vi "LoadGasCalibr.vi"(6 "Enable":bool, 7 "Read":bool, 8 "error in (no error)":errorcluster, 10 "Cluster":T1, 11 "VISA Refnum in":refnum<visa-resource-name>) -> (0 "error out":errorcluster, 1 "Array Graph":cluster{u16[], u16[]}[](array[cluster]), 3 "Array INT":i32[][](array[numeric]))   [LabVIEW 2020]
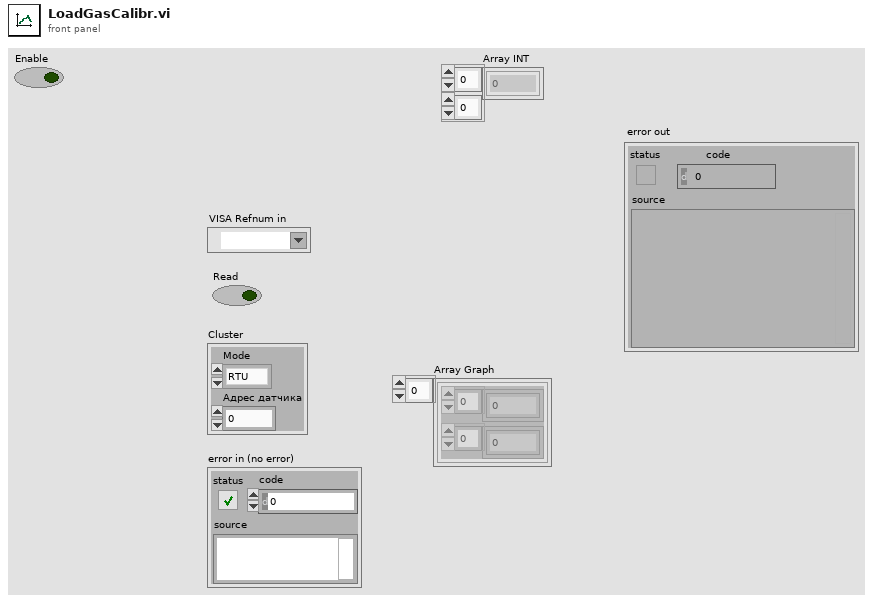
[diagram p1: front panel]
types:
  T1 = cluster{"Mode":enum16{"RTU", "ASCII"}, "Адрес датчика":u16}
  T2 = cluster{"Mode":enum16{"RTU", "ASCII"}, "Новый адрес датчика":u16}
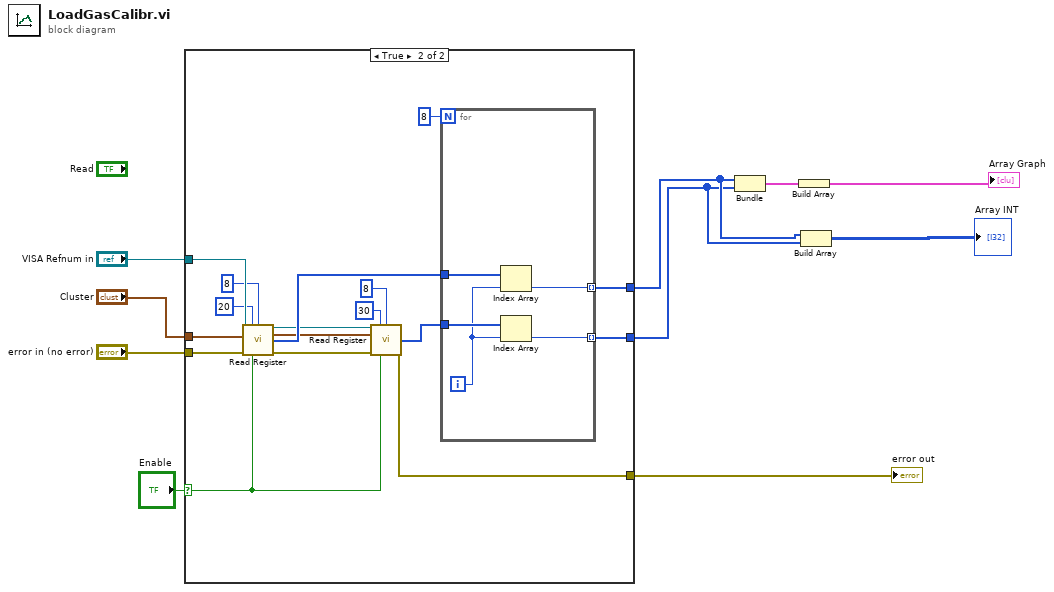
[diagram p0: block diagram]
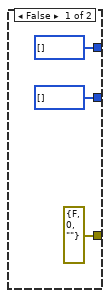
[diagram p2: hidden frame]
diagram:
  n1 = case shown="True" "Enable" {
    selector: "Enable" -> [_ w14]
    tunnel: "error in (no error)" -> [_ w24]
    tunnel: "Cluster" -> [_ w23]
    tunnel: "VISA Refnum in" -> [_ w22]
    tunnel: [errorcluster {"status"=FALSE, "code"=0, "source"=""} ("error out") w21] -> w6
    tunnel: [i32[] [] w16] -> w4
    tunnel: [i32[] [] w15] -> w3
    frame False {
    }
    frame True {
      n2 = call "Read Register.vi"("Refnum in"=w22, "startReg"=20 ("x"), "Quantity"=8 ("x"), "Mode"=w23, "error in (no error)"=w24, "Enable"=w14) -> ("Refnum Out"=w26:refnum<visa-resource-name>, "ModeOut"=w27:T2, "Holding Registers"=w29:u16[], "error out"=w25:errorcluster)  [unwired: 5 in, 1 out]
      n3 = call "Read Register.vi"("Refnum in"=w26, "startReg"=30 ("x"), "Quantity"=8 ("x"), "Mode"=w27, "error in (no error)"=w25, "Enable"=w14) -> ("Holding Registers"=w30:u16[], "error out"=w21:errorcluster)  [unwired: 5 in, 3 out]
      n4 = for {
        N: 8 -> [_]
        tunnel: w29 -> [w35]
        tunnel: w30 -> [w34]
        tunnel: [w31] -> w15 mode=indexing
        tunnel: [w32] -> w16 mode=indexing
        i -> [w33]
        n5 = Index Array(array=w35, index=w33) -> (element=w32:u16)
        n6 = Index Array(array=w34, index=w33) -> (element=w31:u16)
      }
    }
  }
  "error out" <- w6
  n7 = Bundle(w4, w3) -> (w7:cluster{i32[], i32[]})  [unwired: 1 in]
  n8 = Build Array(w7) -> (→"Array Graph":cluster{i32[], i32[]}[])
  n9 = Build Array(w4, w3) -> (→"Array INT":i32[][])
